vi "Instantiate.vi"(8 "error in (no error)":errorcluster) -> (0 "error out":errorcluster, 3 "Document out":refnum<class "Document.lvclass">)   [LabVIEW 2016, in "Document.lvclass"]
uses:
  Document.lvclass
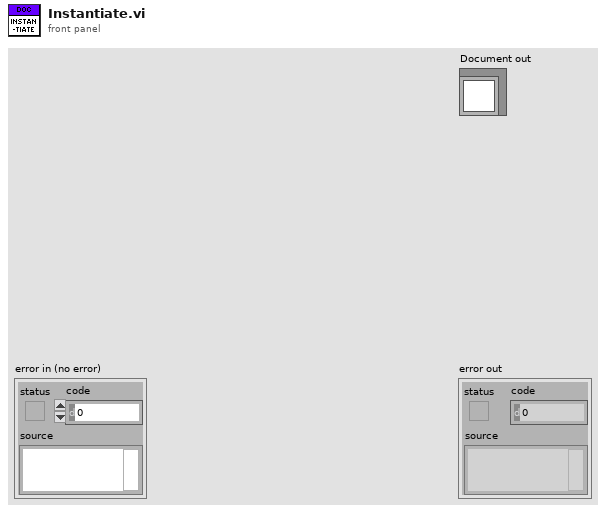
[diagram p1: front panel]
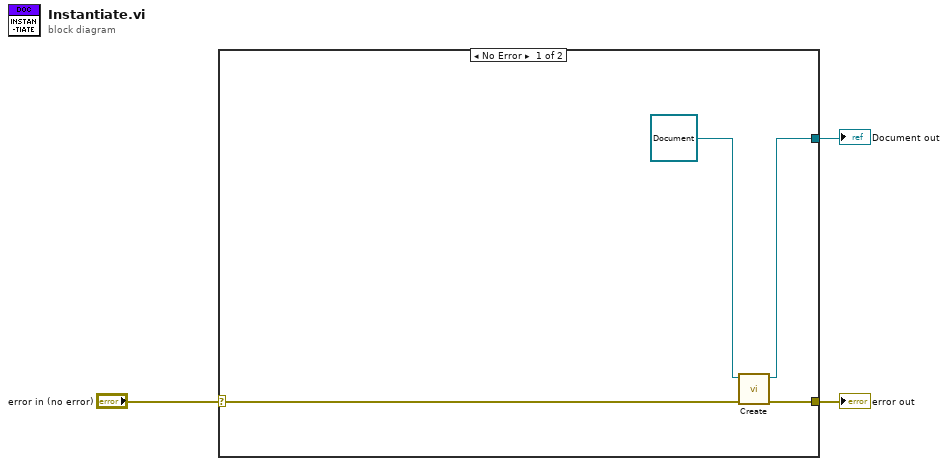
[diagram p0: block diagram]
diagram:
  n1 = case shown="No Error" "error in (no error)" {
    selector: "error in (no error)" -> [w7 w8]
    tunnel: [w6 w8] -> w2
    tunnel: [w4 _] -> w1
    frame No Error {
      n2 = call-dynamic "Create.vi"("error in (no error)"=w7, "Document in"=refnum<class "Document.lvclass"> refnum ("Document out")) -> ("error out"=w6:errorcluster, "Document out"=w4:refnum<class "Document.lvclass">)  [unwired: 8 in]
    }
    frame Error {
    }
  }
  "error out" <- w2
  "Document out" <- w1
